vi "Obtain update control(s) event.vi"(8 "error in (no error)":errorcluster, 11 "Fiber Auto Collimation panel":refnum<class "Fiber Auto Collimation panel.lvclass">) -> (0 "error out":errorcluster, 3 "Update Control(s)":refnum<user-event>)   [LabVIEW 2018, in "Fiber Auto Collimation References.lvclass"]
doc: "This VI gets the reference to an event that should be used only in a view loop to send a signal to itself that it should check for all controls that have been listed as needing to be updated. Because this VI needs to be limited to one panel, it requires a Panel object as an input. If this is on a panel that is cloneable, it needs to be an object with the clone name written to it.\n\nThe data type for this event is a time stamp so that if needed, it can be checked to see if there has been a notable delay between the time the event was requested and the time it actually ran. This is intended to be used for debugging to see if there's a noticible delay between the first request for a control update and the actual control update.\n\nThe event case that this triggers is specially designed to delete all other pending events of the same type but leaving in any other pending events. The actual list of controls is kept separately, and it is recommended that this VI not be used directly to send the event, and only be used to register the event or inside of the \"Send\" VI that was designed to send it.\n\nBecause this event is created once per panel and once per clone, it should be destroyed right before the panel finally closes to avoid memory leaks."
uses:
  Fiber Auto Collimation References.lvclass
  Panels/Fiber Auto Collimation panel.lvclass
  C:/Program Files (x86)/National Instruments/LabVIEW 2018/user.lib/nLight Tidbits/Cross-library references/Cross-library key/Cross-library key.lvclass
  b47026bc-8271-46ff-bcce-21c2580a6587.vi
  f406f5ab-9891-41e2-b0a1-c13e850666b3.vi
  b47026bc-8271-46ff-bcce-21c2580a6587.vi/80a55534-07b4-46f3-95dc-9cfd723c105d.vi
  <userlib>/nLight Tidbits/Cross-library references/Cross-library key/Obtain cross library semaphore and acquire.vi
  b47026bc-8271-46ff-bcce-21c2580a6587.vi/4da48868-7ba5-4708-8795-12157d94ca14.vi
  f406f5ab-9891-41e2-b0a1-c13e850666b3.vi/53d4c5d6-f8c1-450b-89f8-0892ad8fc76d.vi
  f406f5ab-9891-41e2-b0a1-c13e850666b3.vi/861b9ba3-e80f-41d3-82b8-501c193dd8d2.vi
  <userlib>/nLight Error Handling/Trash error.vi
  <vilib>/Utility/error.llb/Clear Errors.vi
  <vilib>/Utility/semaphor.llb/Obtain Semaphore Reference.vi
  <vilib>/Utility/semaphor.llb/Acquire Semaphore.vi
  <userlib>/nLight Error Handling/Log any errors.vi
  <userlib>/nLight Tidbits/Cross-library references/Cross-library key/Obtain class key.vi
  <vilib>/Utility/semaphor.llb/Release Semaphore.vi
  <vilib>/Utility/semaphor.llb/Release Semaphore Reference.vi
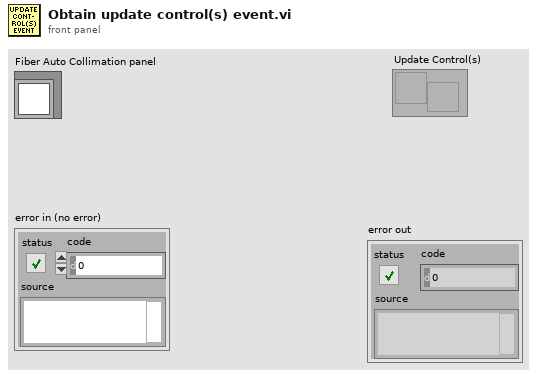
[diagram p1: front panel]
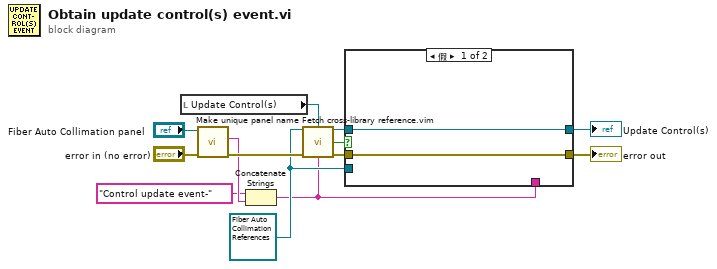
[diagram p0: block diagram]
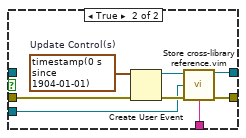
[diagram p2: hidden frame]
diagram:
  w7 = refnum<class "Fiber Auto Collimation References.lvclass"> refnum ("nLight Station Template References.lvclass")
  n1 = local read "Update Control(s)"() -> (w8:refnum<user-event>)
  n2 = call "Make unique panel name.vi"("error in (no error)"="error in (no error)", "Fiber Auto Collimation panel in"="Fiber Auto Collimation panel") -> ("error out"=w9:errorcluster, "Unique panel name"=w3:string)  [unwired: 7 in, 1 out]
  n3 = Concatenate Strings("Control update event-" ("string"), w3) -> (w2:string)
  n4 = call "Fetch cross-library reference.vim"("Cross-library key"=w7, "Reference type to fetch"=w8, "error in (no error)"=w9, "Specific ref type name [String/Enum]"=w2) -> ("Stored value (if present)"=w4:refnum<user-event>, "Nothing to fetch OR bad reference"=w6:bool, "error out"=w5:errorcluster)  [unwired: 9 in]
  n5 = case shown="假" w6 {
    tunnel: w5 -> [w14 w23]
    tunnel: [w14 w18] -> w12
    tunnel: [w15 w19] -> w13
    tunnel: w4 -> [w15 _]
    tunnel: w7 -> [_ w17]
    tunnel: w2 -> [_ w16]
    frame False {
    }
    frame True {
      w22 = timestamp(0 s since 1904-01-01)  # Update Control(s)
      n6 = Create User Event(user event datatype=w22, error in=w23) -> (user event=w20:refnum<user-event>, error out=w21:errorcluster)
      n7 = call "Store cross-library reference.vim"("Reference to store"=w20, "Cross-library key"=w17, "error in (no error)"=w21, "Specific ref type name [String/Enum]"=w16) -> ("Copy of stored reference"=w19:refnum<user-event>, "error out"=w18:errorcluster)  [unwired: 8 in, 2 out]
    }
  }
  "error out" <- w12
  "Update Control(s)" <- w13
